vi "save_scan_settings.vi"(8 "Path":path, 10 "New scan settings":T1={"Start voltage (V)"=0.0, "End voltage (V)"=1.4, "Number of steps"=0, "Settling delay (ms)"=1.4, "Dual sweep"=0, "Stabilisation time (s)"=10.0, "Stabilisation mode"=0, "Stabilisation value (V or A) "=0.0, "No. of repeat scans"=0.0, "Repeat scans"=0, "Logarithmic sweep"=0, "Electrode configuration"=0, "Sweep mode"=0, "Auto settling delay"=1, "Pulse off time (ms)"=0.0, "Integration time (ms)"=1.0, "Current range"=0, "Enable display"=0, "Enable concurrent measurements"=1, "Concurrent measurements"=1} {"Concurrent measurements" items=["Volts", "Current", "Resistance", "Volt, Current", "Volts, Resistance", "Current, Resistance", "All"]; "Enable concurrent measurements" items=["False", "True"]; "Enable display" items=["False", "True"]; "Current range" items=["Auto", "1 uA", "10 uA", "100 uA", "1 mA", "10 mA", "100 mA", "1 A"]; "Integration time (ms)" min=0.2 max=200.0; "Pulse off time (ms)" min=0.0; "Auto settling delay" items=["False", "True"]; "Sweep mode" items=["Staircase", "Pulsed"]; "Electrode configuration" items=["2-wire", "4-wire"]; "Logarithmic sweep" items=["False", "True"]; "Repeat scans" items=["False", "True"]; "No. of repeat scans" min=1.0 step=1.0; "Stabilisation mode" items=["V", "I"]; "Dual sweep" items=["False", "True"]; "Settling delay (ms)" min=0.0 max=999999.9}, 11 "New name":string) -> (0 "error out":errorcluster)   [LabVIEW 2016]
uses:
  TypeDefs/settings.ctl
  <vilib>/Utility/file.llb/Write Delimited Spreadsheet (string).vi
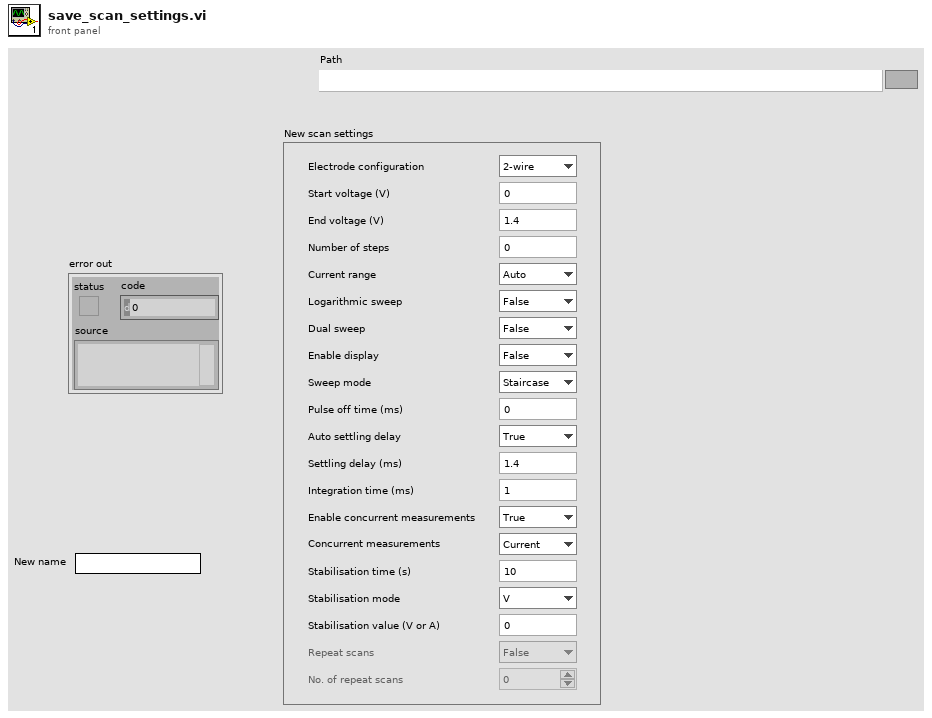
[diagram p1: front panel]
types:
  T1 = typedef "settings.ctl" = cluster{"Start voltage (V)":dbl, "End voltage (V)":dbl, "Number of steps":u32, "Settling delay (ms)":dbl, "Dual sweep":u16, "Stabilisation time (s)":dbl, "Stabilisation mode":u16, "Stabilisation value (V or A) ":dbl, "No. of repeat scans":dbl, "Repeat scans":u16, "Logarithmic sweep":u16, "Electrode configuration":u16, "Sweep mode":u16, "Auto settling delay":u16, "Pulse off time (ms)":dbl, "Integration time (ms)":dbl, "Current range":u16, "Enable display":u16, "Enable concurrent measurements":u16, "Concurrent measurements":u16}
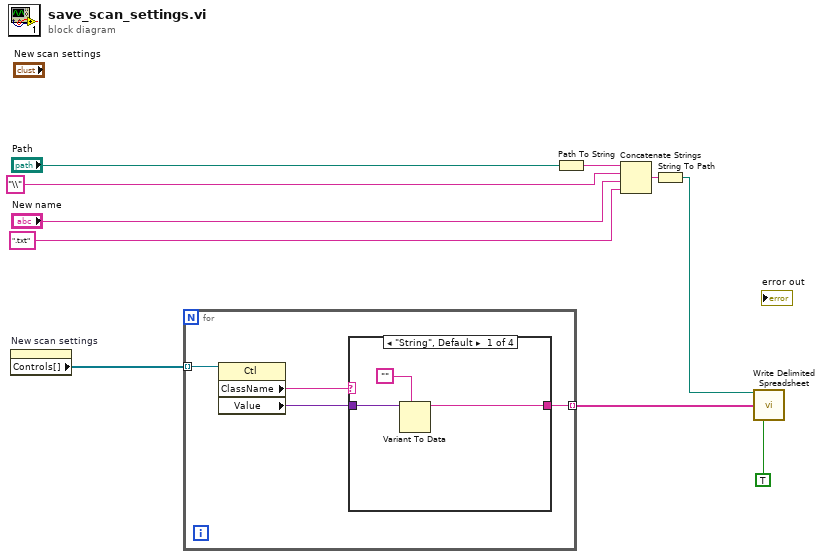
[diagram p0: block diagram]
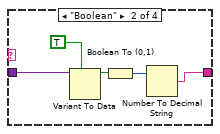
[diagram p2: hidden frame]
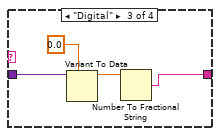
[diagram p3: hidden frame]
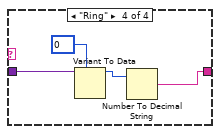
[diagram p4: hidden frame]
diagram:
  n1 = property on="New scan settings" class="Clust (strict)"() -> ("Controls[]"=w4:refnum<vi>[])  [unwired: 2 in, 2 out]
  n2 = for {
    tunnel: w4 -> [w14] mode=indexing
    tunnel: [w11] -> w1 mode=indexing
    n3 = property class="Ctl"(reference=w14) -> ("ClassName"=w13:string, "Value"=w12:variant)  [unwired: 1 in, 2 out]
    n4 = case shown="\"String\", Default" w13 {
      tunnel: w12 -> [w17 w22 w26 w28]
      tunnel: [w15 w18 w23 w27] -> w11
      frame "String", Default {
        n5 = Variant To Data(type="", Variant=w17) -> (data=w15:string)  [unwired: 1 in, 1 out]
      }
      frame "Boolean" {
        n6 = Variant To Data(type=TRUE, Variant=w22) -> (data=w20:bool)  [unwired: 1 in, 1 out]
        n7 = Boolean To (0,1)(Boolean=w20) -> (0, 1=w19:i16)
        n8 = Number To Decimal String(number=w19) -> (decimal integer string=w18:string)  [unwired: 1 in]
      }
      frame "Digital" {
        n9 = Variant To Data(type=0.0, Variant=w26) -> (data=w24:dbl)  [unwired: 1 in, 1 out]
        n10 = Number To Fractional String(number=w24) -> (F-format string=w23:string)  [unwired: 3 in]
      }
      frame "Ring" {
        w30 = u16 0 items=[""]
        n11 = Variant To Data(type=w30, Variant=w28) -> (data=w29:u16)  [unwired: 1 in, 1 out]
        n12 = Number To Decimal String(number=w29) -> (decimal integer string=w27:string)  [unwired: 1 in]
      }
    }
  }
  n13 = Path To String(path="Path") -> (string=w10:string)
  n14 = Concatenate Strings(w10, "\\", "New name", ".txt" ("y")) -> (w9:string)
  n15 = String To Path(string=w9) -> (path=w3:path)
  n16 = call-poly <vilib>:"Write Delimited Spreadsheet.vi"("file path (dialog if empty)"=w3, "1D data"=w1, "transpose? (no:F)"=TRUE) -> ()  [unwired: 11 in, 2 out]
